vi "周期设置_CODMn.vi"() -> ()   [LabVIEW 2016, in "斯坦道CODMn新电路板.lvlib"]
uses:
  <vilib>/Utility/miscctls.llb/LVPointTypeDef.ctl
  <vilib>/Utility/config.llb/NI_LVConfig.lvlib
  <vilib>/ptbypt/NI_PtbyPt.lvlib
panel:
  in  "运行周期":T1={"运行模式"=enum."维护模式", "质控频次"=enum."关闭", "空白核查时间"=2, "跨度核查时间"=6, "测量间隔"=240} {"跨度核查时间" items=["00H", "01H", "02H", "03H", "04H", "05H", "06H", "07H", "08H", "09H", "10H", "11H", "12H", "13H", "14H", "15H", "16H", "17H", "18H", "19H", "20H", "21H", "22H", "23H", "关闭"]; "空白核查时间" items=["00H", "01H", "02H", "03H", "04H", "05H", "06H", "07H", "08H", "09H", "10H", "11H", "12H", "13H", "14H", "15H", "16H", "17H", "18H", "19H", "20H", "21H", "22H", "23H", "关闭"]}
  # "运行模式："
  # "质控频次："
  # "零点核查时间："
  # "跨度核查时间："
  # "测量间隔："
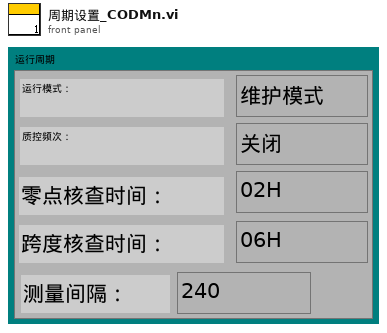
[diagram p1: front panel]
types:
  T1 = cluster{"运行模式":enum16{"维护模式", "常规模式", "应急模式", "质控模式"}, "质控频次":enum16{"关闭", "每天", "星期一", "星期二", "星期三", "星期四", "星期五", "星期六", "星期日"}, "空白核查时间":u16, "跨度核查时间":u16, "测量间隔":u16}
  T2 = typedef "LVPointTypeDef.ctl" = cluster{"Horizontal":i16, "Vertical":i16}
  T3 = typedef "NI_LVConfig.lvlib/Config Data RefNum.ctl" = refnum<k1>
  T4 = enum16{"启动测量", "标样核查", "零点核查", "跨度核查", "空白测试", "平行样测试", "加标回收", "空白校准", "标样校准", "初始化（清洗）", "停止测试", "仪器重启", "校时", "模式设置", "测量间隔设置"}
  T5 = enum16{"关闭", "每天", "星期一", "星期二", "星期三", "星期四", "星期五", "星期六", "星期日"}
  T6 = typedef "LVDateTimeRec.ctl" = cluster{"秒数的小数部分":dbl, "秒":i32, "分":i32, "时":i32, "日":i32, "月":i32, "年":i32, "天数（周）":i32, "天数（年）":i32, "DST":i32}
  T7 = cluster{"运行模式":enum16{"维护模式", "常规模式", "应急模式", "质控模式", "性能测试"}, "质控频次":enum16{"关闭", "每天", "星期一", "星期二", "星期三", "星期四", "星期五", "星期六", "星期日"}, "空白核查时间":u16, "跨度核查时间":u16, "测量间隔":u16}
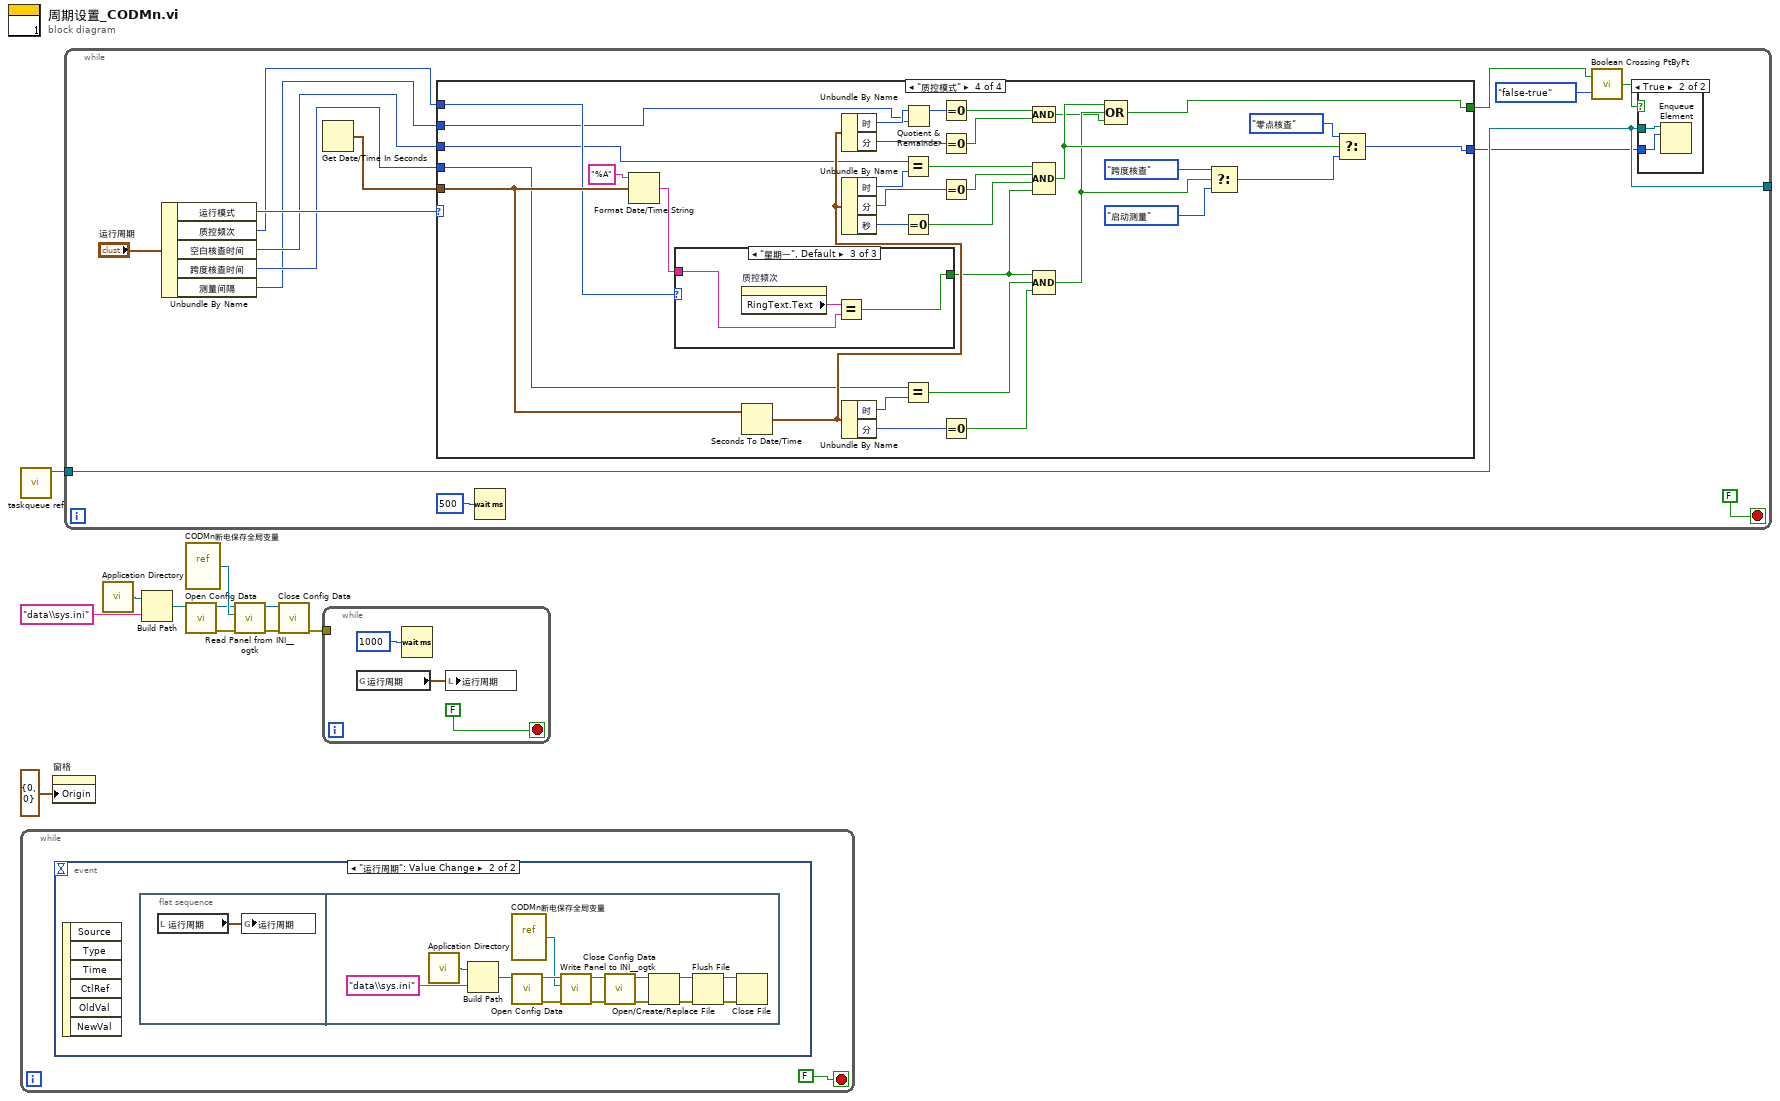
[diagram p0: block diagram]
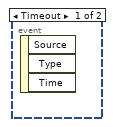
[diagram p2: hidden frame]
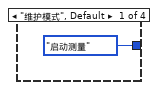
[diagram p4: hidden frame]
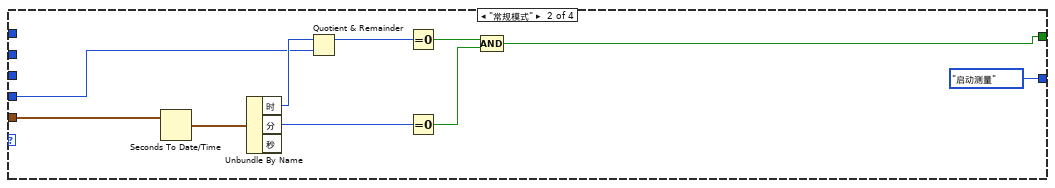
[diagram p5: hidden frame]
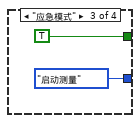
[diagram p6: hidden frame]
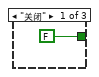
[diagram p7: hidden frame]
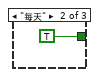
[diagram p8: hidden frame]
diagram:
  n1 = call "taskqueue ref.vi"() -> ("队列输出"=w1:refnum<queue>)  [unwired: 10 in, 1 out]
  n2 = while {
    stop <- FALSE stop-if-true
    n3 = event shown="[1] \"运行周期\": Value Change" {
      selector: _ -> [_ _]
      dyn-events: _ -> [_ _]
      timeout: _ -> [_ _]
      event Timeout {
        n4 = event-data() -> ()  [unwired: 1 in, 3 out]
      }
      event "运行周期": Value Change {
        n5 = event-data() -> ()  [unwired: 1 in, 6 out]
        n6 = flat-sequence {
          frame #0 {
            n7 = local read "运行周期"() -> (w13:T1)
            n8 = global write "CODMn断电保存全局变量.vi" "运行周期"(w13) -> ()
          }
          frame #1 {
            n9 = call <vilib>:"Application Directory.vi"() -> ("Application Directory"=w27:path)
            n10 = Build Path(base path=w27, name or relative path="data\\sys.ini" ("名称或相对路径")) -> (appended path=w25:path)
            n11 = vi-ref "CODMn断电保存全局变量.vi"() -> (w23:refnum<vi>)
            n12 = call <vilib>:"Open Config Data.vi"("configuration file path"=w25) -> ("error out"=w21:errorcluster, "refnum"=w24:T3)  [unwired: 8 in, 1 out]
            n13 = call <userlib>:"Write Panel to INI__ogtk.vi"("error in (no error)"=w21, "VI ref"=w23, "refnum"=w24) -> ("error out"=w20:errorcluster, "refnum out"=w22:T3)  [unwired: 7 in]
            n14 = call <vilib>:"Close Config Data.vi"("error in (no error)"=w20, "refnum"=w22) -> ("error out"=w15:errorcluster, "file path"=w14:path)  [unwired: 8 in]
            n15 = Open/Create/Replace File(file path (use dialog)=w14, error in=w15) -> (refnum out=w18:refnum<file>, error out=w19:errorcluster)  [unwired: 4 in, 1 out]
            n16 = Flush File(refnum=w18, error in=w19) -> (refnum out=w17:refnum<file>, error out=w16:errorcluster)
            n17 = Close File(refnum=w17, error in=w16) -> ()  [unwired: 2 out]
          }
        }
      }
    }
  }
  n18 = property on="窗格" class="Pane"("Origin"=T2 {"Horizontal"=0, "Vertical"=0} ("原点")) -> ()  [unwired: 2 in, 2 out]
  n19 = while {
    tunnel: [w33] -> _
    tunnel: w1 -> [w33]
    stop <- FALSE stop-if-true
    n20 = Unbundle By Name("运行周期") -> ("运行模式"=w38:enum16{"维护模式", "常规模式", "应急模式", "质控模式"}, "质控频次"=w37:T5, "空白核查时间"=w36:u16, "跨度核查时间"=w35:u16, "测量间隔"=w34:u16)
    n21 = Get Date/Time In Seconds() -> (seconds since 1Jan1904=w41:timestamp)
    n22 = case shown="\"质控模式\"" w38 {
      tunnel: w41 -> [_ w54 _ w89]
      tunnel: w34 -> [_ _ _ w59]
      tunnel: [_ w50 TRUE w73] -> w31
      tunnel: [T4."启动测量" ("控制命令") T4."启动测量" ("控制命令") T4."启动测量" ("控制命令") w69] -> w32
      tunnel: w37 -> [_ _ _ w66]
      tunnel: w36 -> [_ _ _ w65]
      tunnel: w35 -> [_ w47 _ w64]
      frame "维护模式", Default {
      }
      frame "常规模式" {
        n23 = Seconds To Date/Time(time stamp (now)=w54) -> (date time rec=w53:T6)  [unwired: 1 in]
        n24 = Unbundle By Name(w53) -> ("时"=w48:i32, "分"=w52:i32)  [unwired: 1 out]
        n25 = Quotient & Remainder(x=w48, y=w47) -> (x-y*floor(x/y)=w46:i32)  [unwired: 1 out]
        n26 = Equal To 0?(x=w46) -> (x = 0?=w45:bool)
        n27 = Equal To 0?(x=w52) -> (x = 0?=w51:bool)
        n28 = Compound Arithmetic op=AND ("复合运算")(w45, w51) -> (w50:bool)
      }
      frame "应急模式" {
      }
      frame "质控模式" {
        n29 = Format Date/Time String(time format string (%c)="%A" ("时间格式字符串(%c)"), seconds (now)=w89) -> (date/time string=w87:string)  [unwired: 1 in]
        n30 = case shown="\"星期一\", Default" w66 {
          tunnel: w87 -> [_ _ w94]
          tunnel: [FALSE TRUE w93] -> w67
          frame "关闭" {
          }
          frame "每天" {
          }
          frame "星期一", Default {
            n31 = property on="质控频次" class="Enum (strict)"() -> ("RingText.Text"=w92:string)  [unwired: 2 in, 2 out]
            n32 = Equal?(x=w92, y=w94) -> (x = y?=w93:bool)
          }
        }
        n33 = Seconds To Date/Time(time stamp (now)=w89) -> (date time rec=w76:T6)  [unwired: 1 in]
        n34 = Unbundle By Name(w76) -> ("时"=w60:i32, "分"=w86:i32)
        n35 = Unbundle By Name(w76) -> ("时"=w84:i32, "分"=w83:i32, "秒"=w82:i32)
        n36 = Unbundle By Name(w76) -> ("时"=w77:i32, "分"=w78:i32)
        n37 = Equal?(x=w65, y=w84) -> (x = y?=w81:bool)
        n38 = Equal To 0?(x=w82) -> (x = 0?=w79:bool)
        n39 = Equal?(x=w64, y=w77) -> (x = y?=w75:bool)
        n40 = Quotient & Remainder(x=w60, y=w59) -> (x-y*floor(x/y)=w58:i32)  [unwired: 1 out]
        n41 = Equal To 0?(x=w58) -> (x = 0?=w57:bool)
        n42 = Equal To 0?(x=w86) -> (x = 0?=w85:bool)
        n43 = Equal To 0?(x=w83) -> (x = 0?=w80:bool)
        n44 = Equal To 0?(x=w78) -> (x = 0?=w74:bool)
        n45 = Compound Arithmetic op=AND ("复合运算")(w57, w85) -> (w68:bool)
        n46 = Compound Arithmetic op=AND ("复合运算")(w81, w80, w79, w67) -> (w72:bool)
        n47 = Compound Arithmetic op=AND ("复合运算")(w67, w75, w74) -> (w71:bool)
        n48 = Compound Arithmetic op=OR ("复合运算")(w72, w71, w68) -> (w73:bool)
        n49 = Select(t=T4."跨度核查" ("控制命令"), s=w71, f=T4."启动测量" ("控制命令")) -> (s? t:f=w70:T4)
        n50 = Select(t=T4."零点核查" ("控制命令"), s=w72, f=w70) -> (s? t:f=w69:T4)
      }
    }
    n51 = Wait (ms)(milliseconds to wait=u32 500 ("等待时间（毫秒）")) -> ()  [unwired: 1 out]
    n52 = call <vilib>:"Boolean Crossing PtByPt.vi"("direction"=enum16{"either", "false-true", "true-false"}."false-true", "input"=w31) -> ("crossing"=w29:bool)  [unwired: 1 in]
    n53 = case shown="True" w29 {
      tunnel: w33 -> [_ w43]
      tunnel: w32 -> [_ w42]
      frame False {
      }
      frame True {
        n54 = Enqueue Element(queue=w43, element=w42) -> ()  [unwired: 2 in, 3 out]
      }
    }
  }
  n55 = call <vilib>:"Application Directory.vi"() -> ("Application Directory"=w4:path)
  n56 = Build Path(base path=w4, name or relative path="data\\sys.ini" ("名称或相对路径")) -> (appended path=w6:path)
  n57 = vi-ref "CODMn断电保存全局变量.vi"() -> (w8:refnum<vi>)
  n58 = call <vilib>:"Open Config Data.vi"("configuration file path"=w6) -> ("error out"=w10:errorcluster, "refnum"=w7:T3)  [unwired: 8 in, 1 out]
  n59 = call <userlib>:"Read Panel from INI__ogtk.vi"("error in (no error)"=w10, "VI ref"=w8, "refnum"=w7) -> ("error out"=w11:errorcluster, "refnum out"=w9:T3)  [unwired: 7 in]
  n60 = call <vilib>:"Close Config Data.vi"("error in (no error)"=w11, "refnum"=w9) -> ("error out"=w3:errorcluster)  [unwired: 8 in, 1 out]
  n61 = while {
    tunnel: w3 -> [_]
    stop <- FALSE stop-if-true
    n62 = global read "CODMn断电保存全局变量.vi" "运行周期"() -> (w95:T7)
    n63 = Wait (ms)(milliseconds to wait=u32 1000 ("等待时间（毫秒）")) -> ()  [unwired: 1 out]
    n64 = local write "运行周期"(w95) -> ()
  }
